vi "GetDeviceInfo.vi"(8 "error in (no error)":errorcluster, 11 "USB-9215 in":refnum<class "USB-9215.lvclass">) -> (0 "error out":errorcluster, 1 "MaxSampleClock":dbl, 2 "ChannelCount":dbl, 3 "USB-9215 out":refnum<class "USB-9215.lvclass">, 5 "DeviceName":string)   [LabVIEW 2013, in "USB-9215.lvclass"]
uses:
  USB-9215.lvclass
  DAQSuper/DAQSuper.lvclass
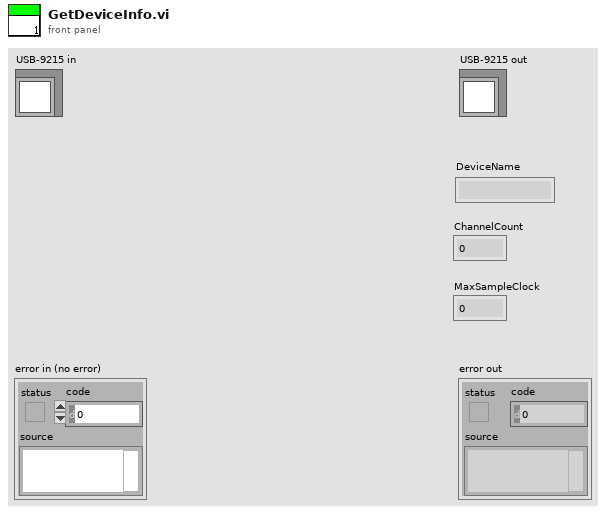
[diagram p1: front panel]
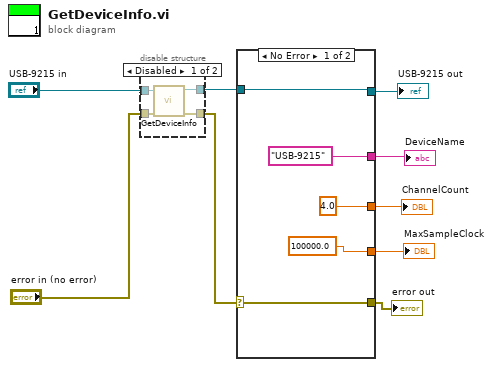
[diagram p0: block diagram]
diagram:
  n1 = disable-structure shown="Disabled" {
    disable-tunnel: [w13 w14] -> w7
    disable-tunnel: [w12 w15] -> w4
    disable-tunnel: "error in (no error)" -> [w11 w14]
    disable-tunnel: "USB-9215 in" -> [w10 w15]
    frame Disabled {
      n2 = call-parent "GetDeviceInfo.vi"("error in (no error)"=w11, "DAQSuper in"=w10) -> ("error out"=w13:errorcluster, "DAQSuper out"=w12:refnum<class "USB-9215.lvclass">)  [unwired: 5 in, 3 out]
    }
    frame Enabled {
    }
  }
  n3 = case shown="No Error" w7 {
    selector: w7 -> [w20 w22]
    tunnel: [w20 w22] -> w6
    tunnel: [w19 w21] -> w5
    tunnel: w4 -> [w19 w21]
    tunnel: [100000.0 _] -> w3
    tunnel: [4.0 _] -> w2
    tunnel: ["USB-9215" _] -> w1
    frame No Error {
    }
    frame Error {
    }
  }
  "error out" <- w6
  "USB-9215 out" <- w5
  "DeviceName" <- w1
  "ChannelCount" <- w2
  "MaxSampleClock" <- w3
